vi "main_fp.vi"() -> ()   [LabVIEW 2016]
uses:
  <vilib>/Instr/_visa.llb/Select Event Type.ctl
  <vilib>/Utility/error.llb/DialogType.ctl
  <vilib>/Platform/TimedLoop/XDataNode/timing_clust.ctl
  <vilib>/Platform/TimedLoop/XDataNode/nitl_modes.ctl
  <vilib>/Platform/TimedLoop/XDataNode/wakeup.ctl
  <vilib>/httpClient/ClientHandle.ctl
  <vilib>/platform/TimedLoop/XDataNode/XDataNode.xnode
  <vilib>/httpClient/LabVIEWHTTPClient.lvlib
  <vilib>/Platform/TimedLoop/XDataNode/XDNodeRunTimeDep.lvlib
panel:
  in  "Tab Control 2":enum32{"Graph panel ¹1", "Current temperature"}(tab)
  out "Waveform Chart":T1(graph)
  out "Internet OK":bool
  in  "VISA resource name":refnum<visa-resource-name>
  out "Status panel of sensors #1":T2
  in  "Remove Button":bool
  out "Temperature sensor #4,°C":dbl(knob) scale=0.0..100.0
  out "Temperature sensor #3,°C":dbl(knob) scale=0.0..100.0
  out "Temperature sensor #2,°C":dbl(knob) scale=0.0..100.0
  out "Temperature sensor #1,°C":dbl(knob) scale=0.1..100.0
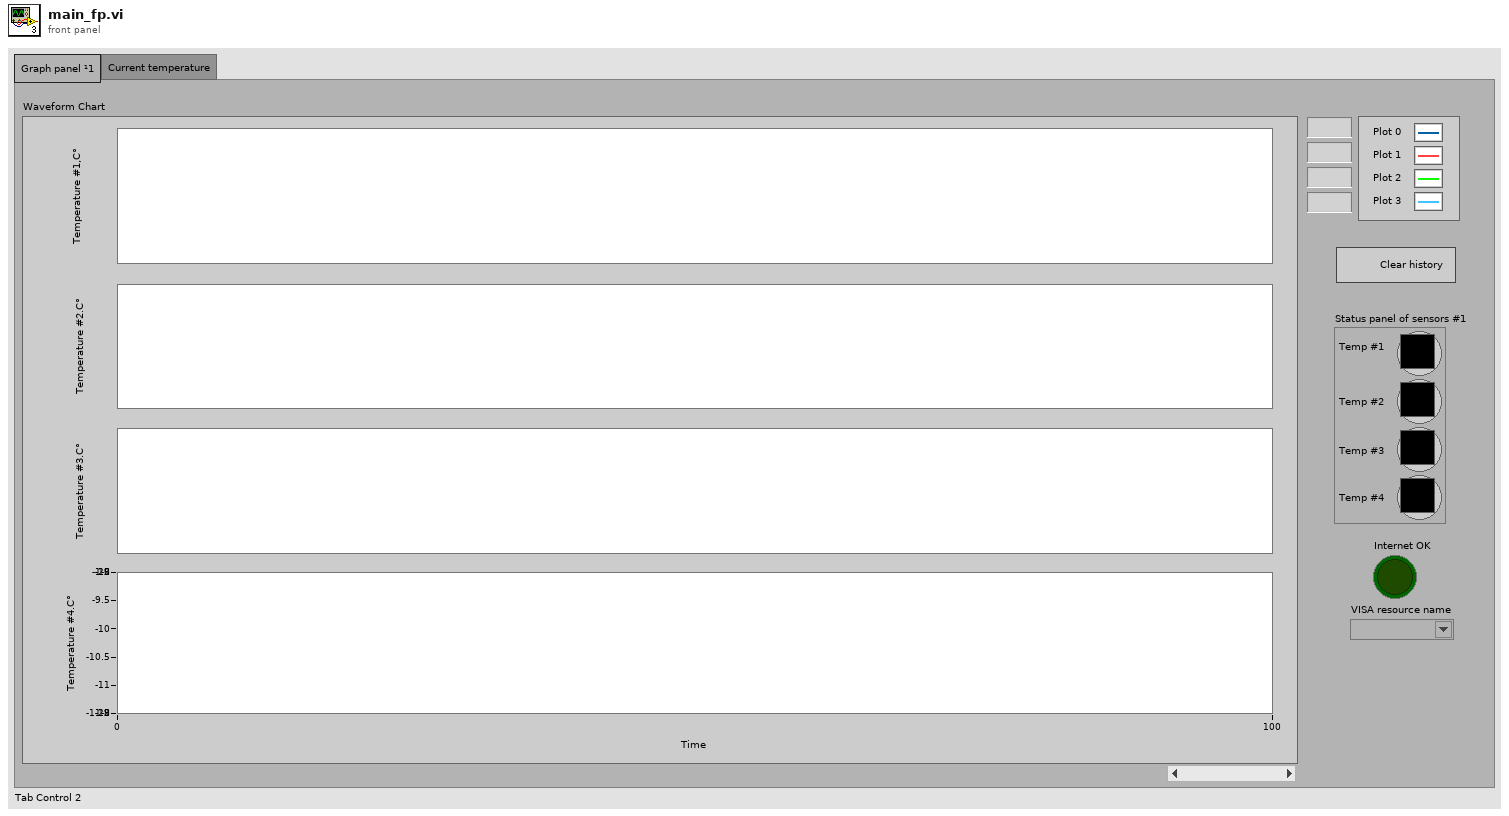
[diagram p1: front panel]
types:
  T1 = cluster{"[0]":dbl, "[1]":dbl, "[2]":dbl, "[3]":dbl}
  T2 = cluster{"Temp #1":u32, "Temp #2":u32, "Temp #3":u32, "Temp #4":u32}
  T3 = typedef "DialogType.ctl" = u16
  T4 = typedef "Select Event Type.ctl" = u32
  T5 = typedef "LabVIEWHTTPClient.lvlib/ClientHandle.ctl" = refnum<k1>
  T6 = typedef "XDNodeRunTimeDep.lvlib/timing_clust.ctl" = cluster{"Expected End [f-1]":u64, "Actual End [f-1]":u64, "Finished Late? [f-1]":bool, "Expected End [i-1]":u64, "Actual End [i-1]":u64, "Finished Late? [i-1]":bool, "Expected Start [i]":u64, "Actual Start [i]":u64, "Expected Start [f]":u64, "Actual Start [f]":u64, "Source Name":string, "Structure Name":string, "Period":i64, "Deadline":i64, "Offset":i64, "Start":i64, "Priority":i32, "Timeout":i32, "Mode":T7, "Wakeup Reason":T8, "Error":errorcluster, "Source Type":string, "Secondary Source Type":string, "Global End Time":u64, "Global Start Time":u64, "Frame Duration":u64, "Iteration Duration":u64, "Assigned CPU":i32, "I/O Scan Engine Mode":u32}
  T7 = typedef "XDNodeRunTimeDep.lvlib/nitl_modes.ctl" = enum32{"No Change", "Process missed periods, maintain original phase", "Discard missed periods, maintain original phase", "Process missed periods, ignore original phase", "Discard missed periods, ignore original phase"}
  T8 = typedef "XDNodeRunTimeDep.lvlib/wakeup.ctl" = enum32{"Normal", "Aborted", "Asynchronous wakeup", "Timing source error", "Timed loop error", "Timeout"}
  T9 = cluster{"[0]":u32, "[1]":u32, "[2]":u32, "[3]":u32}
  T10 = cluster{"client":cluster{"andr_output_volt":dbl}}
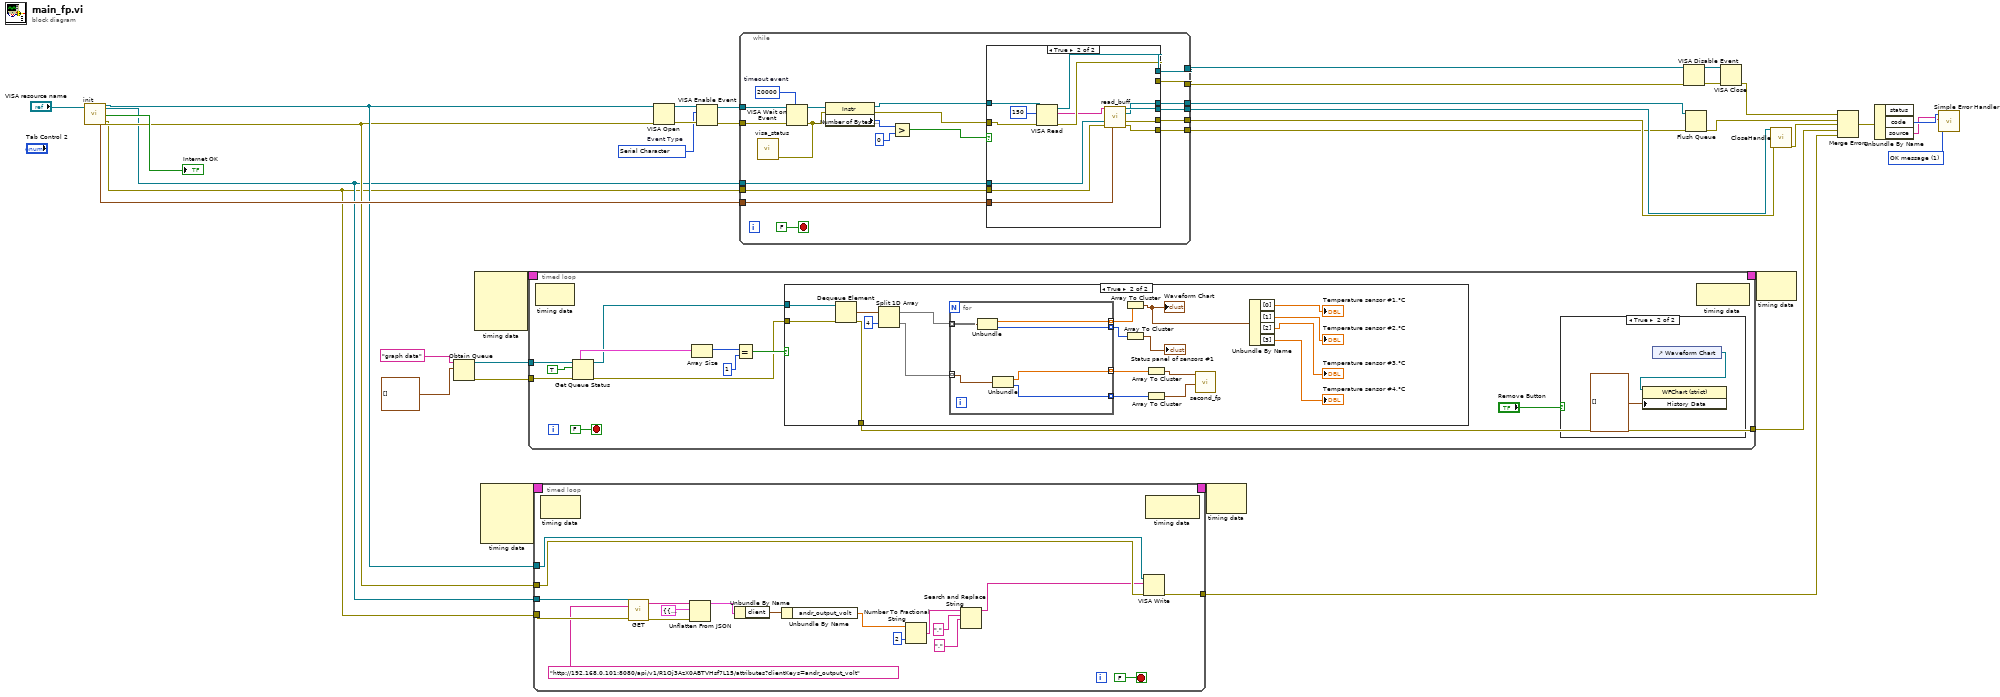
[diagram p0: block diagram]
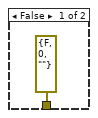
[diagram p3: hidden frame]
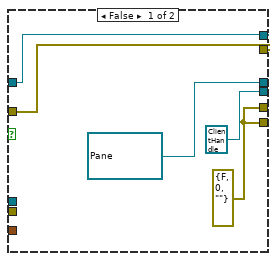
[diagram p4: hidden frame]
diagram:
  w17 = T3 1 items=["no dialog", "OK message", "continue or stop message", "OK message + warnings", "continue/stop + warnings"] ("type of dialog (OK msg:1)")
  w31 = T4 1073684533 items=["Service Request"=1073684491, "Trigger"=3221168138, "Clear"=1073684493, "VXI Signal"=1073684512, "VXI/VME Interrupt"=3221168161, "VXI/VME Sysfail"=1073684509, "VXI/VME Sysreset"=1073684510, "GPIB CIC"=1073684498, "GPIB Talk"=1073684499, "GPIB Listen"=1073684500, "PXI Interrupt"=1073684514, "Serial Break"=1073684515, "Serial TermChar"=1073684516, "Serial CTS"=1073684521, "Serial DSR"=1073684522, "Serial DCD"=1073684524, "Serial RI"=1073684526, "Serial Character"=1073684533, "USB Interrupt"=1073684535, "All Enabled"=1073709055]  # Event Type
  n1 = call "init.vi"("VISA Refnum in"="VISA resource name") -> ("array of ranges"=w15:cluster{"low":dbl, "high":dbl}[], "VISA out"=w5:refnum<visa-resource-name>, "HTTP client handle out"=w3:T5, "Internet OK"=→"Internet OK":bool, "HTTP client error out"=w2:errorcluster, "VISA error out"=w4:errorcluster)  [unwired: 21 in]
  n2 = Obtain Queue(name (unnamed)="graph data", element data type=cluster{dbl, "Round Color Box":u32}[] []) -> (queue out=w10:refnum<queue>, error out=w11:errorcluster)  [unwired: 3 in, 1 out]
  n3 = node-c288() -> (w13:T6)  [unwired: 4 in]
  n4 = node-c288() -> (w7:T6)  [unwired: 4 in]
  n5 = timed-loop {
    tunnel: [w45] -> w9
    timing: w13 -> [_]
    timing-out: [_] -> w12
    tunnel: w11 -> [w42]
    tunnel: w10 -> [w41]
    stop <- FALSE stop-if-true
    n6 = node-c288() -> ()  [unwired: 1 in, 1 out]
    n7 = Get Queue Status(queue=w41, return elements? (F)=TRUE, error in (no error)=w42) -> (queue out=w39:refnum<queue>, error out=w40:errorcluster, elements=w43:cluster{cluster{dbl, "Round Color Box":u32}[]}[])  [unwired: 5 out]
    n8 = Array Size(array=w43) -> (size(s)=w48:i32)
    n9 = Equal?(x=w48, y=1) -> (x = y?=w46:bool)
    n10 = case shown="True" w46 {
      tunnel: w40 -> [_ w62]
      tunnel: [errorcluster {"status"=FALSE, "code"=0, "source"=""} ("error out") w61] -> w45
      tunnel: w39 -> [_ w60]
      frame False {
      }
      frame True {
        n11 = Dequeue Element(queue=w60, error in (no error)=w62) -> (element=w73:cluster{dbl, "Round Color Box":u32}[], error out=w61:errorcluster)  [unwired: 1 in, 2 out]
        n12 = Split 1D Array(array=w73, index=4) -> (first subarray=w71:cluster{dbl, "Round Color Box":u32}[], second subarray=w63:cluster{dbl, "Round Color Box":u32}[])
        n13 = for {
          tunnel: w71 -> [w79] mode=indexing
          tunnel: [w78] -> w69 mode=indexing
          tunnel: [w77] -> w70 mode=indexing
          tunnel: [w76] -> w65 mode=indexing
          tunnel: [w75] -> w64 mode=indexing
          tunnel: w63 -> [w74] mode=indexing
          n14 = Unbundle(w79) -> (w77:dbl, "Round Color Box"=w78:u32)
          n15 = Unbundle(w74) -> (w76:dbl, "Round Color Box"=w75:u32)
        }
        n16 = Array To Cluster(array=w70) -> (cluster=w59:T1)
        "Waveform Chart" <- w59
        n17 = Array To Cluster(array=w69) -> (cluster=→"Status panel of sensors #1":T9)
        n18 = Array To Cluster(array=w65) -> (cluster=w68:T1)
        n19 = Array To Cluster(array=w64) -> (cluster=w67:T9)
        n20 = call "second_fp.vi"("Waveform chart data"=w68, "Stat of sensors"=w67) -> ()  [unwired: 18 in]
        n21 = Unbundle By Name(w59) -> ("[0]"=→"Temperature sensor #1,°C":dbl, "[1]"=→"Temperature sensor #2,°C":dbl, "[2]"=→"Temperature sensor #3,°C":dbl, "[3]"=→"Temperature sensor #4,°C":dbl)
      }
    }
    n22 = case shown="True" "Remove Button" {
      frame False {
      }
      frame True {
        n23 = control-ref of="Waveform Chart"() -> (w52:refnum<vi>)
        n24 = property on="Property Node" class="WFChart (strict)"(reference=w52, "History Data"=cluster{dbl, dbl, dbl, dbl}[] []) -> ()  [unwired: 1 in, 2 out]
      }
    }
    n25 = node-c288() -> ()  [unwired: 1 in, 1 out]
  }
  n26 = timed-loop {
    timing: w7 -> [_]
    timing-out: [_] -> w6
    tunnel: w5 -> [w88]
    tunnel: w4 -> [w87]
    tunnel: w3 -> [w95]
    tunnel: w2 -> [w96]
    tunnel: [w86] -> w1
    stop <- FALSE stop-if-true
    n27 = node-c288() -> ()  [unwired: 1 in, 1 out]
    n28 = call <vilib>:"GET.vi"("client handle"=w95, "url"="http://192.168.0.101:8080/api/v1/R1Oj3AzX0ABTVHsf7L15/attributes?clientKeys=andr_output_volt", "error in (no error)"=w96) -> ("body"=w93:string, "error out"=w84:errorcluster)  [unwired: 9 in, 2 out]
    n29 = Unflatten From JSON(JSON string=w93, type and defaults=T10 {"client"={"andr_output_volt"=0.0}}, error in (no error)=w84) -> (value=w82:T10)  [unwired: 4 in, 1 out]
    n30 = Unbundle By Name(w82) -> ("client"=w81:cluster{"andr_output_volt":dbl})
    n31 = Unbundle By Name(w81) -> ("andr_output_volt"=w80:dbl)
    n32 = Number To Fractional String(number=w80, precision (6)=i16 2) -> (F-format string=w89:string)  [unwired: 2 in]
    n33 = Search and Replace String(input string=w89, search string=",", replace string="." ("replace string (\"\")")) -> (result string=w85:string)  [unwired: 5 in, 3 out]
    n34 = VISA Write(VISA resource name=w88, write buffer=w85, error in (no error)=w87) -> (error out=w86:errorcluster)  [unwired: 2 out]
    n35 = node-c288() -> ()  [unwired: 1 in, 1 out]
  }
  n36 = VISA Open(error in (no error)=w4, VISA resource name=w5) -> (VISA resource name=w37:refnum<visa-resource-name>, error out=w36:errorcluster)  [unwired: 3 in]
  n37 = VISA Enable Event(8:w36, 10:w31, 11:w37) -> (0:w34:errorcluster, 3:w35:refnum<visa-resource-name>)  [unwired: 1 in]
  n38 = while {
    tunnel: w35 -> [w119]
    tunnel: w34 -> [w111]
    tunnel: [w109] -> w30
    tunnel: [w108] -> w8
    tunnel: w3 -> [w106]
    tunnel: w2 -> [w105]
    tunnel: [w104] -> w27
    tunnel: [w103] -> w25
    tunnel: [w102] -> w24
    tunnel: [w101] -> w23
    tunnel: w15 -> [w100]
    stop <- FALSE stop-if-true
    w112 = u32 20000  # timeout event
    n39 = VISA Wait on Event(7:w112, 8:w111, 11:w119) -> (0:w110:errorcluster, 3:w118:refnum<visa-resource-name>)  [unwired: 2 in, 2 out]
    n40 = call "visa_status.vi"("error in (no error)"=w110) -> ()  [unwired: 11 in]
    n41 = property class="Instr"(reference=w118, error in=w110) -> (reference out=w117:refnum<visa-resource-name>, error out=w113:errorcluster, "Serial Settings:Number of Bytes at Serial Port"=w116:u32)
    n42 = Greater?(x=w116, y=u32 0) -> (0:w114:bool)
    n43 = case shown="True" w114 {
      tunnel: w117 -> [w124 w136]
      tunnel: w113 -> [w123 w135]
      tunnel: [w124 w134] -> w109
      tunnel: [w123 w133] -> w108
      tunnel: w106 -> [_ w131]
      tunnel: w105 -> [_ w130]
      tunnel: [w122 w128] -> w104
      tunnel: [T5 refnum ("client handle out") w129] -> w103
      tunnel: [refnum<queue> refnum ("queue out") w127] -> w102
      tunnel: [w122 w126] -> w101
      tunnel: w100 -> [_ w125]
      frame False {
        w122 = errorcluster {"status"=FALSE, "code"=0, "source"=""} ("error queue out")
      }
      frame True {
        n44 = VISA Read(VISA resource name=w136, byte count=u32 150, error in (no error)=w135) -> (VISA resource name out=w134:refnum<visa-resource-name>, read buffer=w132:string, error out=w133:errorcluster)  [unwired: 1 out]
        n45 = call "read_buff.vi"("buffer"=w132, "HTTP client handle"=w131, "HTTP client error"=w130, "array of ranges"=w125) -> ("client handle out"=w129:T5, "queue out"=w127:refnum<queue>, "http client error out"=w128:errorcluster, "error queue out"=w126:errorcluster)  [unwired: 8 in]
      }
    }
  }
  n46 = node-c288(w6) -> ()  [unwired: 1 out]
  n47 = VISA Disable Event(8:w8, 11:w30) -> (0:w33:errorcluster, 3:w32:refnum<visa-resource-name>)  [unwired: 2 in]
  n48 = Flush Queue(queue=w24, error in (no error)=w23) -> (error out=w22:errorcluster)  [unwired: 2 out]
  n49 = VISA Close(VISA resource name=w32, error in (no error)=w33) -> (error out=w21:errorcluster)
  n50 = node-c288(w12) -> ()  [unwired: 1 out]
  n51 = call <vilib>:"CloseHandle.vi"("client handle"=w25, "error in (no error)"=w27) -> ("error out"=w26:errorcluster)  [unwired: 13 in]
  n52 = Merge Errors(w21, w22, w26, w9, w1) -> (w20:errorcluster)
  n53 = Unbundle By Name(w20) -> ("code"=w19:i32, "source"=w18:string)  [unwired: 1 out]
  n54 = call <vilib>:"Simple Error Handler.vi"("error code (no error:0)"=w19, "error source (\" \")"=w18, "type of dialog (OK msg:1)"=w17) -> ()  [unwired: 2 in, 5 out]
